vi "mqttCmdCreate.vi"(8 "error in (no error)":errorcluster, 10 "messageID":u16) -> (0 "error out":errorcluster, 3 "mqttCmdPublishComplete out":refnum<class "mqttCmdPublishComplete.lvclass">)   [LabVIEW 2020, in "mqttCmdPublishComplete.lvclass"]
uses:
  mqttCmdPublishComplete.lvclass
  C:/Projects/Libraries/Gore SM 2020/mqtt-LabVIEW/src/class/mqtt/mqttCmd/mqttCmd.lvclass
  mqttTypedef/mqttMessageType.ctl
  mqttTypedef/mqttQOSlevel.ctl
  mqttCmd.lvclass/mqttCmd.ctl
  Properties/Write Datagram.vi
  mqttCmd.lvclass
  mqtt.lvclass
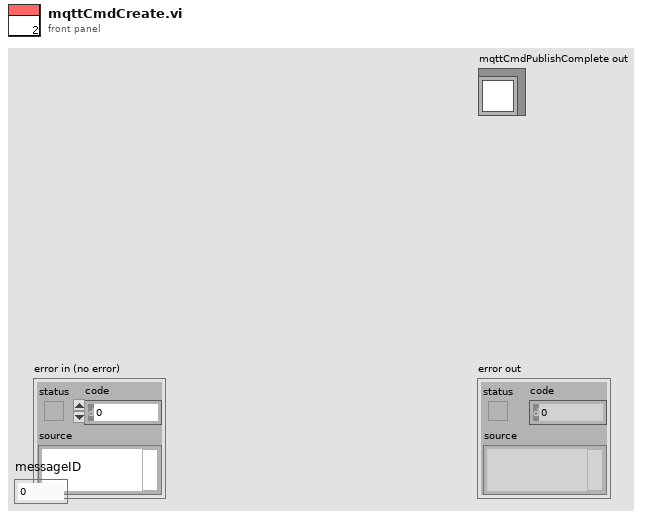
[diagram p1: front panel]
types:
  T1 = typedef "mqtt.lvclass/mqttQOSlevel.ctl" = enum8{"At most once", "At least once", "Exactly once", "Reserved"}
  T2 = typedef "mqtt.lvclass/mqttMessageType.ctl" = enum32{"Reserved", "CONNECT", "CONNACK", "PUBLISH", "PUBACK", "PUBREC", "PUBREL", "PUBCOMP", "SUBSCRIBE", "SUBACK", "UNSUBSCRIBE", "UNSUBACK", "PINGREQ", "PINGRESP", "DISCONNECT", "Reserved2"}
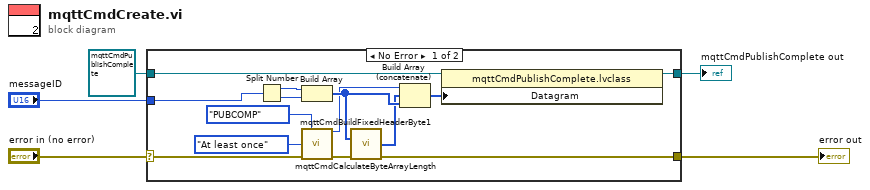
[diagram p0: block diagram]
diagram:
  n1 = case shown="No Error" "error in (no error)" {
    selector: "error in (no error)" -> [w7 w21]
    tunnel: [w8 w21] -> w4
    tunnel: [w10 w20] -> w2
    tunnel: refnum<class "mqttCmdPublishComplete.lvclass"> refnum ("mqttCmdPublishComplete in") -> [w12 w20]
    tunnel: "messageID" -> [w6 _]
    frame No Error {
      n2 = Split Number(x=w6) -> (hi(x)=w16:u8, lo(x)=w15:u8)
      n3 = Build Array(w16, w15) -> (w17:u8[])
      n4 = call "mqttCmdBuildFixedHeaderByte1.vi"("MessageType"=mqttMessageType."PUBCOMP", "QoS (At most once)"=mqttQOSlevel."At least once", "error in (no error)"=w7) -> ("byte1"=w13:u8, "error out"=w9:errorcluster)  [unwired: 11 in]
      n5 = call "mqttCmdCalculateByteArrayLength.vi"("byteArry in"=w17, "error in (no error)"=w9) -> ("length out"=w14:u8[], "error out"=w8:errorcluster)  [unwired: 12 in]
      n6 = Build Array (concatenate)(w13, w14, w17) -> (w11:u8[])
      n7 = property class="mqttCmdPublishComplete.lvclass"(reference=w12, "Datagram"=w11) -> (reference out=w10:refnum<class "mqttCmdPublishComplete.lvclass">)  [unwired: 1 in, 1 out]
    }
    frame Error {
    }
  }
  "error out" <- w4
  "mqttCmdPublishComplete out" <- w2
